vi "initialise.vi"(8 "error in (no error)":errorcluster, 11 "ProEM_WinX32 in":refnum<class "ProEM_WinX32.lvclass">) -> (0 "error out":errorcluster, 3 "ProEM_WinX32 out":refnum<class "ProEM_WinX32.lvclass">)   [LabVIEW 2011, in "Hardware.lvlib" / "Channels.lvlib" / "ProEM_WinX32.lvclass"]
uses:
  ProEM_WinX32.lvclass
  ProEM_WinX32.lvclass/ProEM_WinX32.ctl
  Camera/Camera.lvclass
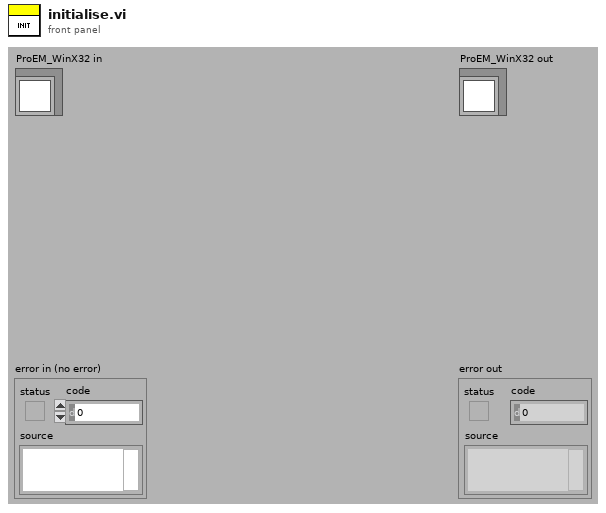
[diagram p1: front panel]
types:
  T1 = cluster{"Message":enum16{"Idle", "initialise", "configureAcquisition", "setTemperature", "getTemperature", "start", "stop", "sendImage", "close", "error", "ExitApp", "getAcquisitionStatus"}, "Data":variant}
  T2 = typedef "WINX32 Object Reference.ctl" = refnum<k1>
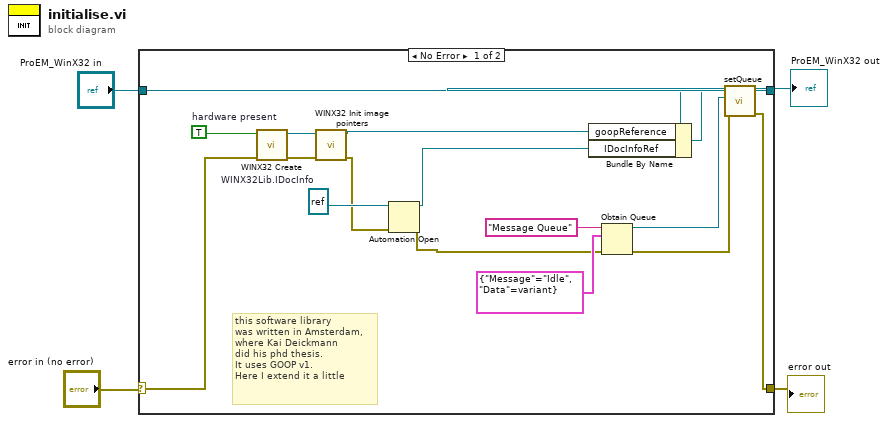
[diagram p0: block diagram]
diagram:
  n1 = case shown="No Error" "error in (no error)" {
    selector: "error in (no error)" -> [w20 w22]
    tunnel: [w12 w23] -> w4
    tunnel: "ProEM_WinX32 in" -> [w19 w23]
    tunnel: [w9 w22] -> w1
    frame No Error {
      w18 = refnum<k7> refnum  # WINX32Lib.IDocInfo
      w21 = TRUE  # hardware present
      # "this software library\nwas written in Amsterdam,\nwhere Kai Deickmann \ndid his phd thesis.\nIt uses GOOP v1.\nHere I extend it a little"
      n2 = call <instrlib>:"WINX32 Create.vi"("error in (no error)"=w20, "hardware present"=w21) -> ("error out"=w7:errorcluster, "reference"=w8:T2)  [unwired: 4 in]
      n3 = call <instrlib>:"WINX32 Init image pointers.vi"("error in (no error)"=w7, "reference"=w8) -> ("error out"=w5:errorcluster, "duplicate reference"=w6:T2)  [unwired: 8 in]
      n4 = Automation Open(error in (no error)=w5, Automation Refnum=w18) -> (Automation Refnum=w17:refnum<k7>, error out=w14:errorcluster)  [unwired: 2 in]
      n5 = Bundle By Name(cluster=w19, "goopReference"=w6, "IDocInfoRef"=w17) -> (w13:refnum<class "ProEM_WinX32.lvclass">)
      n6 = Obtain Queue(name (unnamed)="Message Queue" ("Queue Name"), element data type=T1 {"Message"=enum."Idle", "Data"=variant}, error in (no error)=w14) -> (queue out=w11:refnum<queue>, error out=w10:errorcluster)  [unwired: 2 in, 1 out]
      n7 = call "setQueue.vi"("error in (no error)"=w10, "queue"=w11, "Camera in"=w13) -> ("error out"=w9:errorcluster, "Camera out"=w12:refnum<class "ProEM_WinX32.lvclass">)  [unwired: 7 in]
    }
    frame Error {
    }
  }
  "error out" <- w1
  "ProEM_WinX32 out" <- w4
